vi "odometry.vi"(1 "reset":bool, 2 "distance between sides of wheels":dbl, 3 "encoders in":dbl[](array[numeric]), 4 "state in":dbl[](array[numeric])) -> (0 "state out":dbl[](array[numeric]))   [LabVIEW 2016]
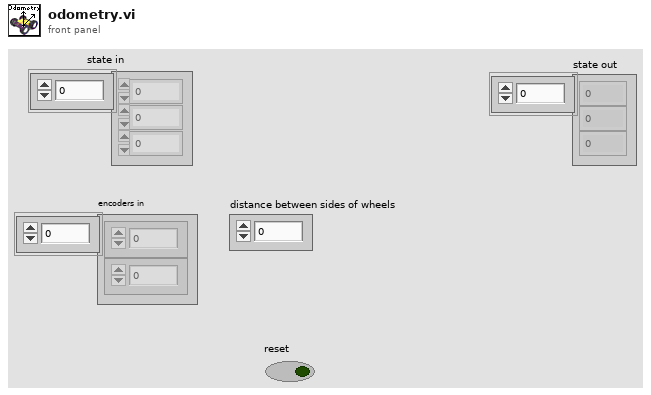
[diagram p1: front panel]
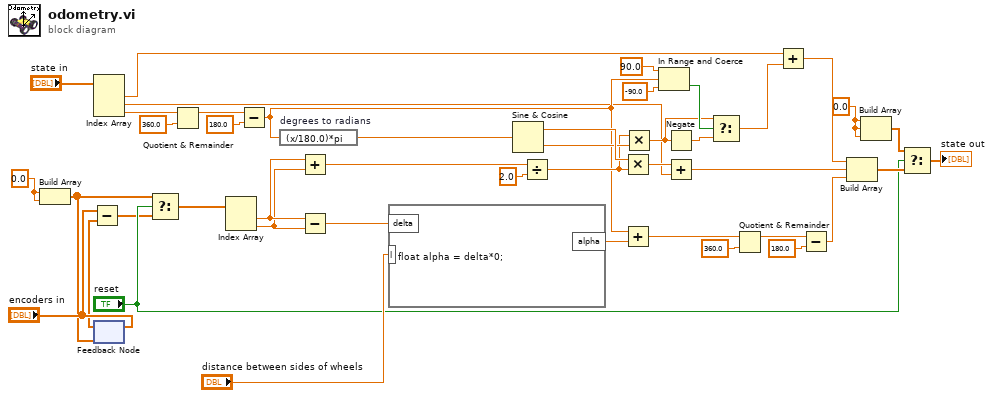
[diagram p0: block diagram]
diagram:
  w4 = 0.0 ("element")
  w11 = 0.0 ("element")
  n1 = Build Array(w11, w11) -> (w5:dbl[])
  n2 = Index Array(array="state in") -> (element #1=w19:dbl, element #2=w18:dbl, element #3=w17:dbl)  [unwired: 3 in]
  n3 = feedback-in #1("encoders in") -> ()
  n4 = feedback #1(w5) -> (w9:dbl[])
  n5 = Subtract(x="encoders in", y=w9) -> (x-y=w2:dbl[])
  n6 = Select(t=w5, s="reset", f=w2) -> (s? t:f=w1:dbl[])
  n7 = Quotient & Remainder(x=w17, y=360.0) -> (x-y*floor(x/y)=w25:dbl)  [unwired: 1 out]
  n8 = Index Array(array=w1) -> (element #1=w13:dbl, element #2=w12:dbl)  [unwired: 2 in]
  n9 = Subtract(x=w25, y=180.0) -> (x-y=w23:dbl)
  n10 = expression code="(x/180.0)*pi" "degrees to radians"(w23) -> (w44:dbl)
  n11 = Add(x=w13, y=w12) -> (x+y=w43:dbl)
  n12 = Subtract(x=w13, y=w12) -> (x-y=w31:dbl)
  n13 = formula code="float alpha = delta*0;"("delta"=w31, "l"="distance between sides of wheels") -> ("alpha"=w29:dbl)
  n14 = Sine & Cosine(0:w44) -> (1:w41:dbl, 2:w40:dbl)
  n15 = Divide(x=w43, y=2.0) -> (x/y=w39:dbl)
  n16 = Multiply(x=w41, y=w39) -> (x*y=w32:dbl)
  n17 = Add(x=w23, y=w29) -> (x+y=w27:dbl)
  n18 = Multiply(x=w39, y=w40) -> (x*y=w34:dbl)
  n19 = In Range and Coerce(upper limit=90.0, x=w23, lower limit=-90.0 ("x")) -> (In Range?=w36:bool)  [unwired: 1 out]
  n20 = Negate(x=w34) -> (-x=w35:dbl)
  n21 = Add(x=w32, y=w18) -> (x+y=w15:dbl)
  n22 = Select(t=w34, s=w36, f=w35) -> (s? t:f=w33:dbl)
  n23 = Quotient & Remainder(x=w27, y=360.0) -> (x-y*floor(x/y)=w21:dbl)  [unwired: 1 out]
  n24 = Add(x=w19, y=w33) -> (x+y=w16:dbl)
  n25 = Subtract(x=w21, y=180.0) -> (x-y=w14:dbl)
  n26 = Build Array(w16, w15, w14) -> (w8:dbl[])
  n27 = Build Array(w4, w4, w4) -> (w3:dbl[])
  n28 = Select(t=w3, s="reset", f=w8) -> (s? t:f=→"state out":dbl[])
